vi "Coordinates check dialogue.vi"() -> (1 "Cancelled":bool)   [LabVIEW 2013]
uses:
  Typedefs/Set Main VI cursor.ctl
  Global Variables/gl_UI Ctrl Refs.vi
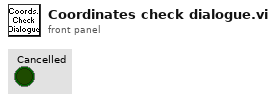
[diagram p1: front panel]
types:
  T1 = typedef "Set Main VI cursor.ctl" = enum16{"Release busy cursor", "Set busy cursor"}
  T2 = enum32{"Basic", "Z-stack ", "Miscellaneous", "Development"}
  T3 = typedef "UI ctrl refs cluster.ctl" = cluster{"Top level VI path":path, "Top level VI ref":refnum<vi>, "User menu ref":refnum<k9>, "Sub Panel control":refnum<vi>, "Imaging Param Tab":refnum<vi>, "Occurrence-Start drivers":refnum<k4>, "Occurrence-Speed logging initialised":refnum<k4>, "Occurrence-XYZ stage initialised":refnum<k4>, "Exit button":refnum<vi>, "Status ind":refnum<vi>, "Return to Origin":refnum<vi>, "Speed Logging":refnum<vi>, "Time Lapse":refnum<vi>, "Live Imaging":refnum<vi>, "AOL Z Stack":refnum<vi>, "Motor Z Stack":refnum<vi>, "Funct Acq button":refnum<vi>, "Hard Shutter":refnum<vi>, "Virtual Shutter":refnum<vi>, "Laser Power":refnum<vi>, "AOL Mode":refnum<vi>, "Frame Size":refnum<vi>, "Field of View":refnum<vi>, "Dwell Time":refnum<vi>, "Zoom":refnum<vi>, "AOL Z":refnum<vi>, "Objective":refnum<vi>, "Axis":refnum<vi>, "Paths & Names":refnum<vi>, "Experiment folder path (ind.)":refnum<vi>, "Last State (Ind.)":refnum<vi>, "Laser wavelength ind (nm)":refnum<vi>, "Averages":refnum<vi>, "Angle (degrees)":refnum<vi>, "X centre":refnum<vi>, "Y centre":refnum<vi>, "Plane Mode":refnum<vi>, "# Planes":refnum<vi>, "Z Start":refnum<vi>, "Z Stop":refnum<vi>, "Z Step":refnum<vi>, "PMT 1":refnum<vi>, "PMT 2":refnum<vi>, "Stage XYZ Position":refnum<vi>, "Pockels@Z Start":refnum<vi>, "Pockels@Z Stop":refnum<vi>, "Obtain Z Start":refnum<vi>, "Obtain Z Stop":refnum<vi>, "Live stim.trig.period":refnum<vi>, "Live stim.trig.enable":refnum<vi>, "Funct. Acq. Pockels Modulation":refnum<vi>, "Enable Video Recording":refnum<vi>, "Video Record-Live Imaging":refnum<vi>, "Video Record-Funct acq":refnum<vi>, "AOL Z-stack Chirps Ready (ind)":refnum<vi>, "Center freq ind (nm)":refnum<vi>, "Logging queue (ind)":refnum<vi>, "Back aperture power (ind.)":refnum<vi>, "Power after objective (ind.)":refnum<vi>, "Switch user":refnum<vi>}
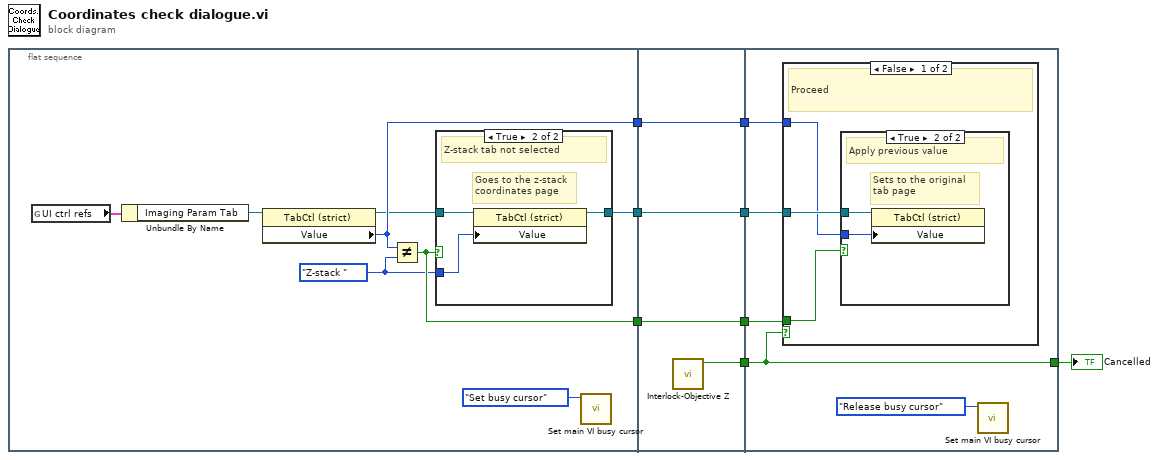
[diagram p0: block diagram]
diagram:
  n1 = flat-sequence {
    tunnel: [w14] -> w5
    tunnel: [w13] -> w3
    tunnel: [w12] -> w2
    tunnel: [w24] -> w7
    tunnel: [w23] -> w6
    tunnel: w5 -> [w23]
    tunnel: [w22] -> w4
    tunnel: w3 -> [w22]
    tunnel: w2 -> [w21]
    tunnel: [w21] -> w1
    tunnel: [w25] -> w8
    tunnel: w7 -> [w25]
    tunnel: w6 -> [w29]
    tunnel: w4 -> [w28]
    tunnel: w1 -> [w27]
    frame #0 {
      w9 = T2."Z-stack " ("Value")
      n2 = global read "gl_UI Ctrl Refs.vi" "UI ctrl refs"() -> (w16:T3)
      n3 = Unbundle By Name(w16) -> ("Imaging Param Tab"=w15:refnum<vi>)
      n4 = property class="TabCtl (strict)"(reference=w15) -> (reference out=w11:refnum<vi>, "Value"=w13:T2)  [unwired: 1 in, 1 out]
      n5 = Not Equal?(x=w13, y=w9) -> (x != y?=w12:bool)
      n6 = case shown="True" w12 {
        tunnel: w11 -> [w17 w19]
        tunnel: [w17 w20] -> w14
        tunnel: w9 -> [_ w18]
        frame False {
          # "Z-stack tab already selected"
        }
        frame True {
          # "Goes to the z-stack\ncoordinates page"
          # "Z-stack tab not selected"
          n7 = property class="TabCtl (strict)"(reference=w19, "Value"=w18) -> (reference out=w20:refnum<vi>)  [unwired: 1 in, 1 out]
        }
      }
      n8 = call "Set main VI busy cursor.vi"("Main VI's cursor"=Set_Main_VI_cursor."Set busy cursor") -> ()  [unwired: 10 in, 1 out]
    }
    frame #1 {
      n9 = call "Interlock-Objective Z.vi"() -> ("Cancelled"=w24:bool)  [unwired: 11 in]
    }
    frame #2 {
      n10 = case shown="False" w25 {
        tunnel: w29 -> [w32 _]
        tunnel: w28 -> [w31 _]
        tunnel: w27 -> [w30 _]
        frame False {
          # "Proceed"
          n11 = case shown="True" w30 {
            tunnel: w32 -> [_ w34]
            tunnel: w31 -> [_ w33]
            frame False {
            }
            frame True {
              # "Sets to the original tab page"
              # "Apply previous value"
              n12 = property class="TabCtl (strict)"(reference=w34, "Value"=w33) -> ()  [unwired: 1 in, 2 out]
            }
          }
        }
        frame True {
          # "User cancelled because they want to make changes to the Z-stack setup values."
        }
      }
      n13 = call "Set main VI busy cursor.vi"("Main VI's cursor"=Set_Main_VI_cursor."Release busy cursor") -> ()  [unwired: 10 in, 1 out]
    }
  }
  "Cancelled" <- w8
